vi "Yokogawa WT1800 Series Acquire Waveform.vi"() -> ()   [LabVIEW 2015]
doc: "This example shows how to use auto ranging and acquire a waveform on a single trace."
uses:
  <instrlib>/Yokogawa WT1800 Series/Public/Configure/Configure Range (Voltage).vi
  <instrlib>/Yokogawa WT1800 Series/Public/Configure/Configure Range (Current 50A).vi
  <instrlib>/Yokogawa WT1800 Series/Public/Data/Read Waveform (Single).vi
  <instrlib>/Yokogawa WT1800 Series/Yokogawa WT1800 Series.lvlib
panel:
  in  "Acquisition Time (50 ms)":dbl(ring)=0.05 items=["0.5m"=0.0005, "1m"=0.001, "2m"=0.002, "5m"=0.005, "10m"=0.01, "20m"=0.02, "50m"=0.05, "100m"=0.1, "200m"=0.2, "500m"=0.5]
  in  "Auto Range (F: Disable)":bool
  in  "Trace (0: U1)":i32(ring) items=["U1", "I1", "U2", "I2", "U3", "I3", "U4", "I4", "U5", "I5", "U6", "I6", "Speed", "Torque", "AUX1", "AUX2"]
  in  "Timeout (10000 ms)":i32=10000 min=1
  in  "VISA resource name":refnum<visa-resource-name>
  out "Waveform Graph":T1(graph)
  # "(c) 2011 Yokogawa Meters & Instruments Corporation.  All rights reserved."
  # "WT1800 SERIES POWER ANALYZER"
  # "s"
  # "ms"
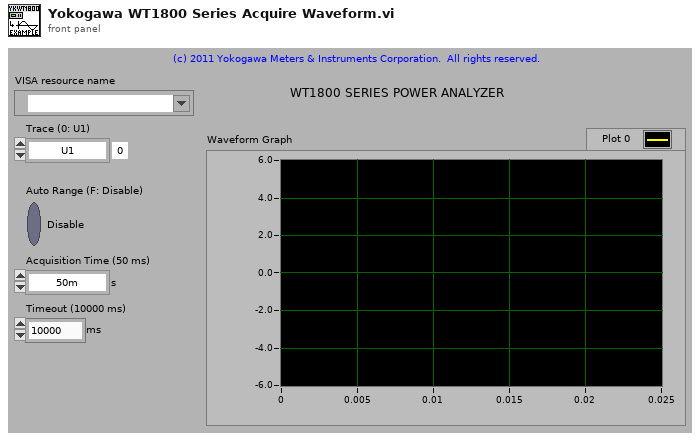
[diagram p1: front panel]
types:
  T1 = cluster{"start":dbl, "Sampling Time":dbl, "Output":dbl[]}
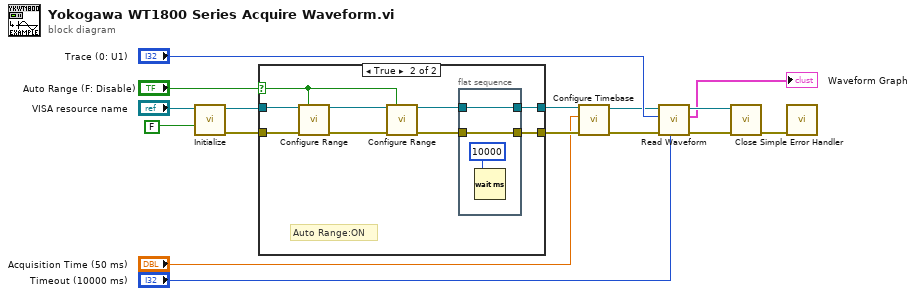
[diagram p0: block diagram]
diagram:
  n1 = call <instrlib>:"Initialize.vi"("Reset (True)"=FALSE, "VISA resource name"="VISA resource name") -> ("error out"=w6:errorcluster, "VISA resource name out"=w7:refnum<visa-resource-name>)  [unwired: 8 in]
  n2 = case shown="True" "Auto Range (F: Disable)" {
    selector: "Auto Range (F: Disable)" -> [_ w19]
    tunnel: w6 -> [w17 w22]
    tunnel: [w17 w27] -> w4
    tunnel: w7 -> [w18 w23]
    tunnel: [w18 w26] -> w5
    frame False {
      # "Auto Range:OFF"
    }
    frame True {
      # "Auto Range:ON"
      n3 = call-poly <instrlib>:"Configure Range.vi"("VISA resource name"=w23, "Auto Range (F: Disable)"=w19, "error in (no error)"=w22) -> ("VISA resource name out"=w24:refnum<visa-resource-name>, "error out"=w25:errorcluster)  [unwired: 11 in]
      n4 = call-poly <instrlib>:"Configure Range.vi"("VISA resource name"=w24, "Auto Range (F: Disable)"=w19, "error in (no error)"=w25) -> ("VISA resource name out"=w21:refnum<visa-resource-name>, "error out"=w20:errorcluster)  [unwired: 11 in]
      n5 = flat-sequence {
        tunnel: [w29] -> w27
        tunnel: w20 -> [w29]
        tunnel: [w28] -> w26
        tunnel: w21 -> [w28]
        frame #0 {
          n6 = Wait (ms)(milliseconds to wait=u32 10000 ("ミリ秒待ち時間")) -> ()  [unwired: 1 out]
        }
      }
    }
  }
  n7 = call <instrlib>:"Configure Timebase.vi"("error in (no error)"=w4, "Acquisition Time (50 ms)"="Acquisition Time (50 ms)", "VISA resource name"=w5) -> ("error out"=w2:errorcluster, "VISA resource name out"=w3:refnum<visa-resource-name>)  [unwired: 7 in]
  n8 = call-poly <instrlib>:"Read Waveform.vi"("Timeout (10000 ms)"="Timeout (10000 ms)", "error in (no error)"=w2, "Trace (0: U1)"="Trace (0: U1)", "VISA resource name"=w3) -> ("error out"=w12:errorcluster, "Waveform Data"=→"Waveform Graph":T1, "VISA resource name out"=w13:refnum<visa-resource-name>)  [unwired: 5 in]
  n9 = call <instrlib>:"Close.vi"("error in (no error)"=w12, "VISA resource name"=w13) -> ("error out"=w11:errorcluster)  [unwired: 9 in]
  n10 = call <vilib>:"Simple Error Handler.vi"("error in (no error)"=w11) -> ()  [unwired: 4 in, 5 out]
